vi "VI.vi"   [LabVIEW 2020]
uses:
  <instrlib>/Agilent 34401/Public/Data/Read (Multiple Points).vi
  <instrlib>/Agilent 2000 3000 X-Series/Public/Data/Read Measurement (Current Value).vi
  <instrlib>/Agilent 34401/Agilent 34401.lvlib
  <instrlib>/Agilent 2000 3000 X-Series/Agilent 2000 3000 X-Series.lvlib
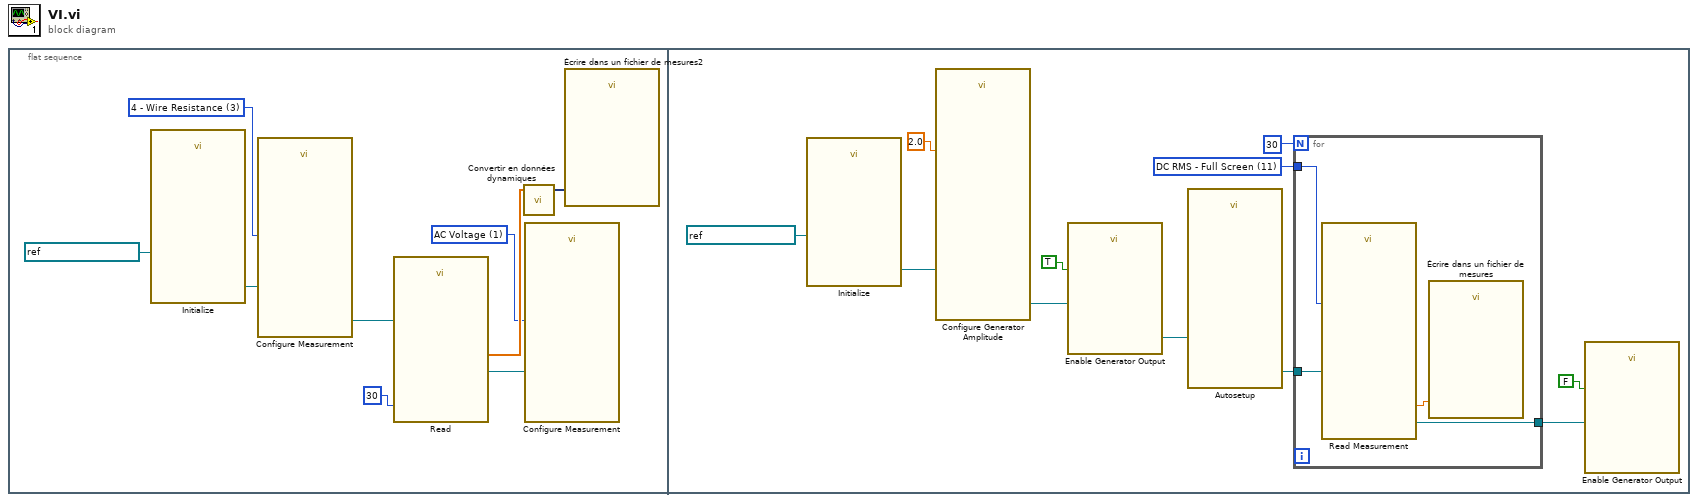
[diagram p0: block diagram]
diagram:
  n1 = flat-sequence {
    frame #0 {
      w4 = u16 1 items=["DC Voltage", "AC Voltage", "2 - Wire Resistance", "4 - Wire Resistance", "DC Current", "AC Current", "Frequency", "Period", "Continuity", "Diode Checking", "VDC:VDC Ratio", "Temperature", "Capacitance"] ("Function (0: DC Voltage)")
      w2 = u16 3 items=["DC Voltage", "AC Voltage", "2 - Wire Resistance", "4 - Wire Resistance", "DC Current", "AC Current", "Frequency", "Period", "Continuity", "Diode Checking", "VDC:VDC Ratio", "Temperature", "Capacitance"] ("Function (0: DC Voltage)")
      n2 = call <instrlib>:"Initialize.vi"("VISA resource name"=refnum<visa-resource-name> "GPIB0::22::INSTR") -> ("VISA resource name out"=w5:refnum<visa-resource-name>)  [unwired: 9 in, 1 out]
      n3 = call <instrlib>:"Configure Measurement.vi"("Function (0: DC Voltage)"=w2, "VISA resource name"=w5) -> ("VISA resource name out"=w6:refnum<visa-resource-name>)  [unwired: 8 in, 1 out]
      n4 = call-poly <instrlib>:"Read.vi"("Sample Count (1)"=30, "VISA resource name"=w6) -> ("Measurements"=w8:dbl[], "VISA resource name out"=w7:refnum<visa-resource-name>)  [unwired: 7 in, 1 out]
      n5 = call "Convertir en données dynamiques"("Array"=w8) -> ("Dynamic Data Type"=w9:dynamicdata)  [unwired: 3 in]
      n6 = call <instrlib>:"Configure Measurement.vi"("Function (0: DC Voltage)"=w4, "VISA resource name"=w7) -> ()  [unwired: 8 in, 2 out]
      n7 = call "Écrire dans un fichier de mesures2"("Signals"=w9) -> ()  [unwired: 16 in, 3 out]
    }
    frame #1 {
      w13 = 11 items=["Peak-Peak", "Maximum", "Mimimum", "Amplitude", "Top", "Base", "Overshoot", "Preshoot", "Average - N Cycles", "Average - Full Screen", "DC RMS - N Cycles", "DC RMS - Full Screen", "AC RMS - N Cycles", "AC RMS - Full Screen (Std Dev)", "Ratio", "Period", "Frequency", "Counter", "+Width", "-Width", "Burst Width", "Duty Cycle", "Rise Time", "Fall Time", "Delay", "Phase", "X minY", "X maxY", "Positive Pulse Count", "Negative Pulse Count", "Raising Edge Count", "Falling Edge Count", "Area - N Cycle", "Area - Full Screen", "Nth Edge Time", "Nth Edge Cross Level Time"] ("Measurement Type (0: Peak-Peak)")
      n8 = call <instrlib>:"Initialize.vi"("VISA resource name"=refnum<visa-resource-name> "GPIB0::7::INSTR") -> ("VISA resource name out"=w16:refnum<visa-resource-name>)  [unwired: 9 in, 1 out]
      n9 = call <instrlib>:"Configure Generator Amplitude.vi"("VISA resource name"=w16, "Amplitude (1.0 V)"=2.0) -> ("VISA resource name out"=w17:refnum<visa-resource-name>)  [unwired: 12 in, 1 out]
      n10 = call <instrlib>:"Enable Generator Output.vi"("Enable Output (F: Disable)"=TRUE, "VISA resource name"=w17) -> ("VISA resource name out"=w18:refnum<visa-resource-name>)  [unwired: 8 in, 1 out]
      n11 = call <instrlib>:"Autosetup.vi"("VISA resource name"=w18) -> ("VISA resource name out"=w19:refnum<visa-resource-name>)  [unwired: 9 in, 1 out]
      n12 = for {
        N: 30 -> [_]
        tunnel: w13 -> [w24]
        tunnel: w19 -> [w23]
        tunnel: [w22] -> w20
        n13 = call-poly <instrlib>:"Read Measurement.vi"("VISA resource name"=w23, "Measurement Type (0: Peak-Peak)"=w24) -> ("VISA resource name out"=w22:refnum<visa-resource-name>, "Result Value"=w21:dbl)  [unwired: 11 in, 1 out]
        n14 = call "Écrire dans un fichier de mesures"("Signals"=w21) -> ()  [unwired: 16 in, 3 out]
      }
      n15 = call <instrlib>:"Enable Generator Output.vi"("Enable Output (F: Disable)"=FALSE, "VISA resource name"=w20) -> ()  [unwired: 8 in, 2 out]
    }
  }
